vi "AWS Credentials Dialog.vi"(8 "error in (no error)":errorcluster) -> (0 "error out":errorcluster, 2 "Secret Access Key":string="fpHFy/9MTHgVK4Kfo+TPLrNeMAvaW8SEbrhzqAeY", 3 "Access Key ID":string="AKIAZ3CRVRJNHJHHHPO3")   [LabVIEW 2016, in "Data.S3.lvclass"]
uses:
  Data.S3/Data.S3.lvclass
  <vilib>/Platform/browser.llb/Open URL in Default Browser (string).vi
panel:
  in  "OK":bool caption="OK1"
  in  "HELP":bool caption="OK1"
  in  "Secret Access Key":string
  in  "Access Key ID":string
  out "String":string="Please enter your AWS credentials below:"
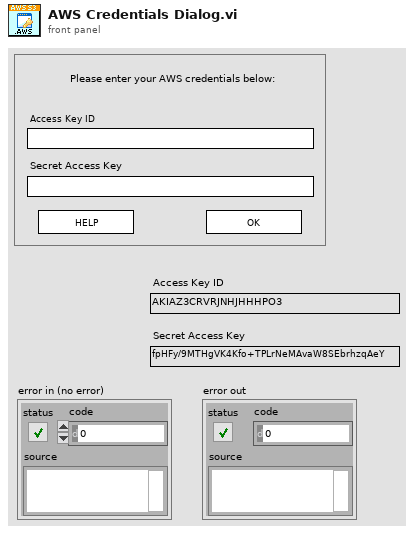
[diagram p1: front panel]
types:
  T1 = enum32{"Invalid", "Standard", "Closed", "Hidden", "Minimized", "Maximized"}
  T2 = enum32{"invalid app kind", "Development System", "Run Time System", "Student Edition", "Embedded LabVIEW", "Evaluation", "Custom"}
  T3 = cluster{"Core":cluster{"Current VI Reference":refnum<vi>, "Close Panel on Exit?":bool}, "Access Key ID":string, "Secret Access Key":string}
  T4 = cluster{"Current VI Reference":refnum<vi>, "Close Panel on Exit?":bool}
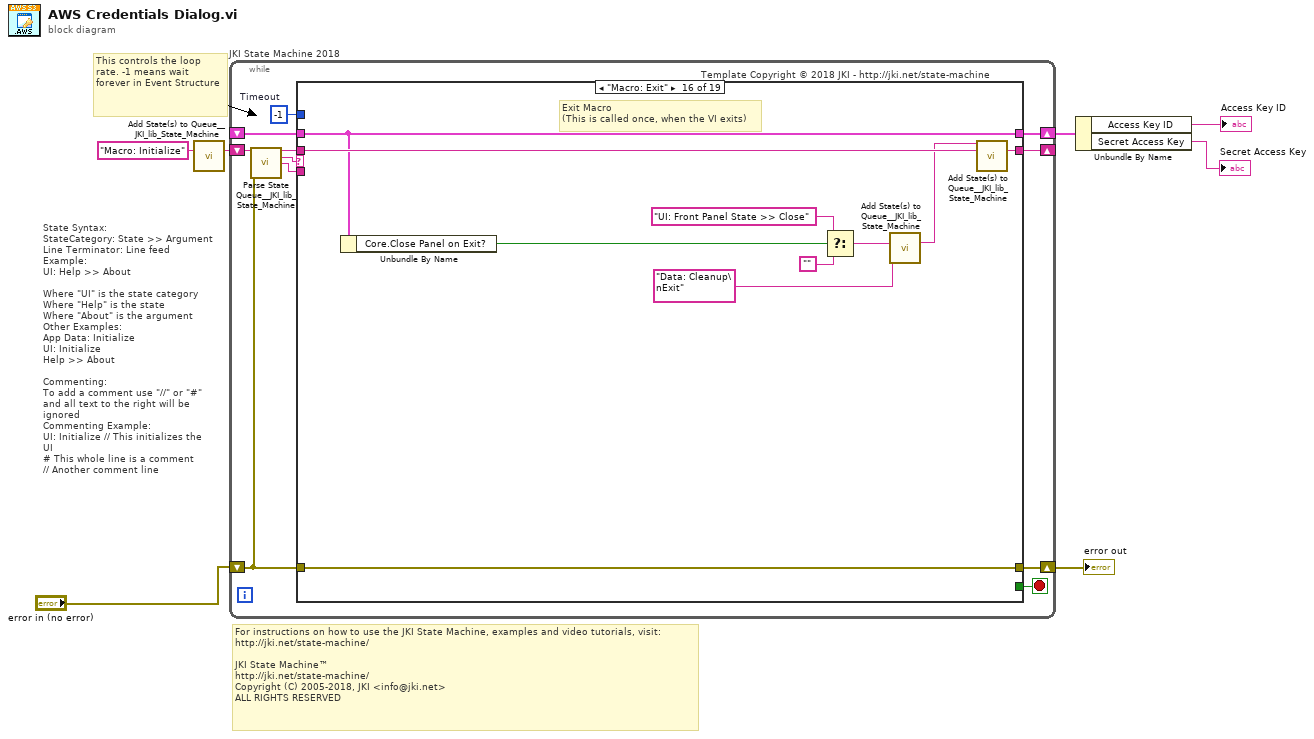
[diagram p0: block diagram]
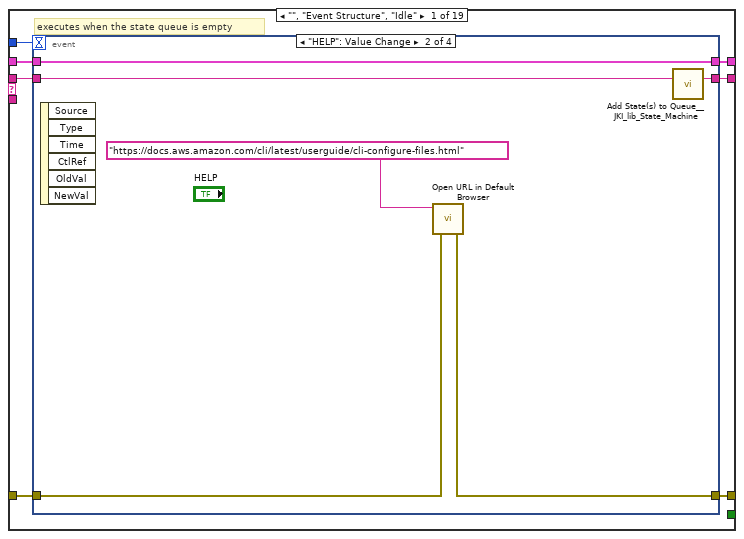
[diagram p2: hidden frame]
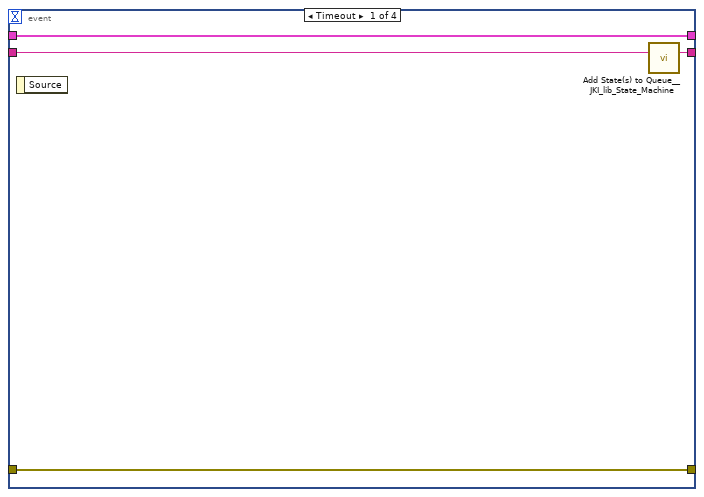
[diagram p3: hidden frame]
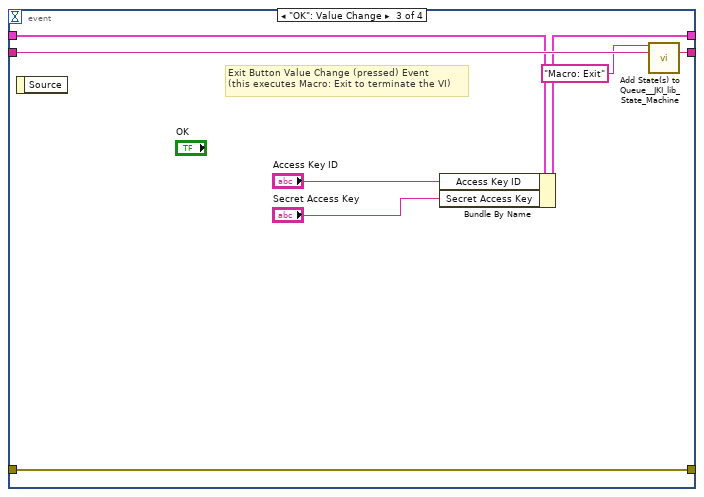
[diagram p4: hidden frame]
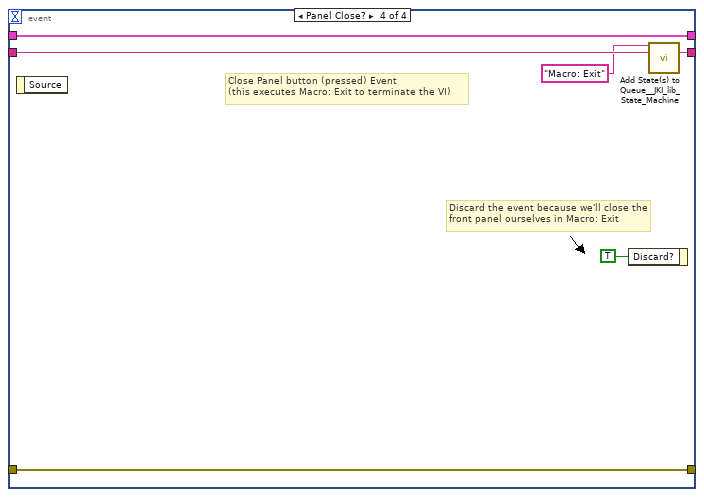
[diagram p5: hidden frame]
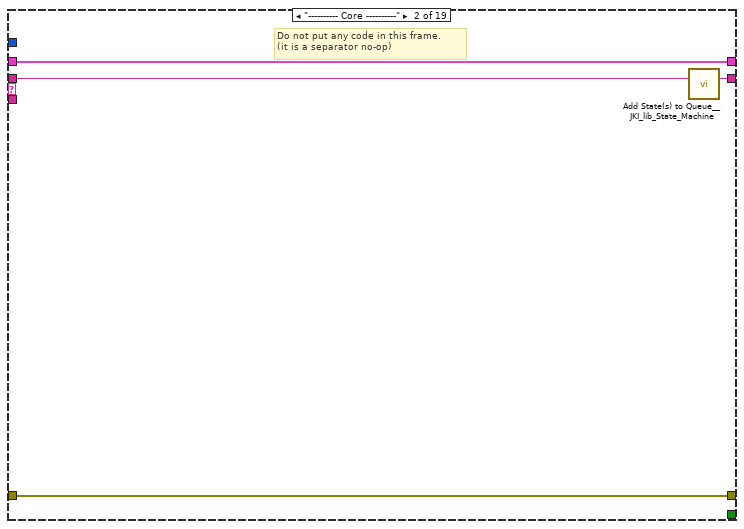
[diagram p6: hidden frame]
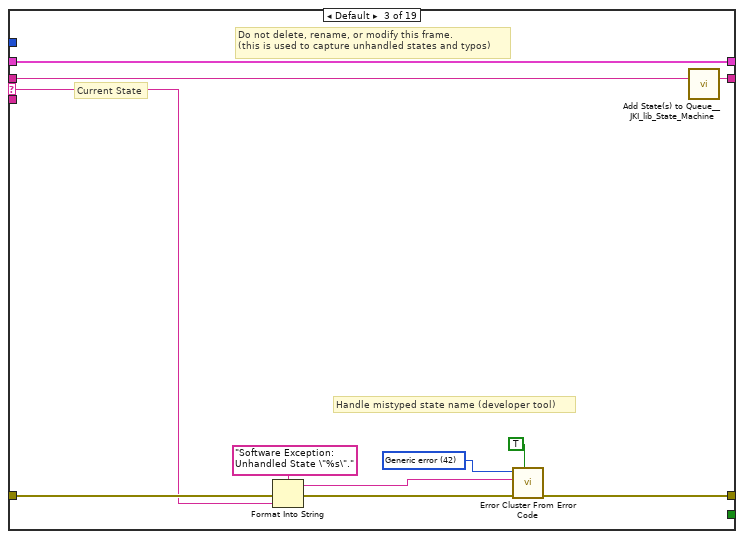
[diagram p7: hidden frame]
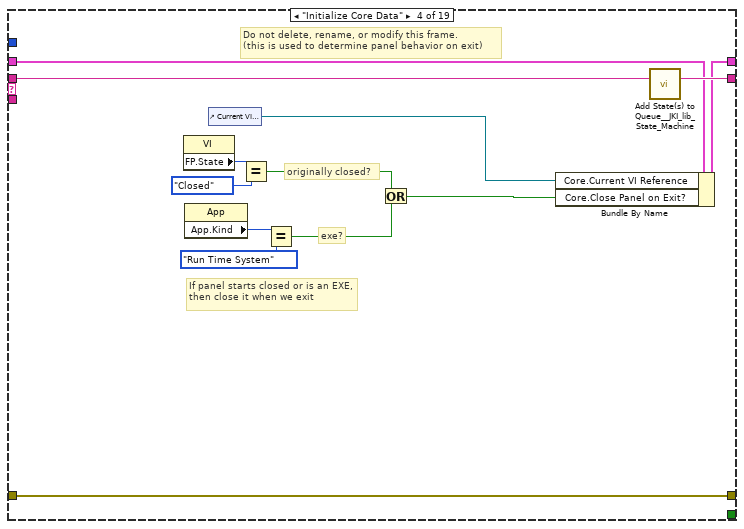
[diagram p8: hidden frame]
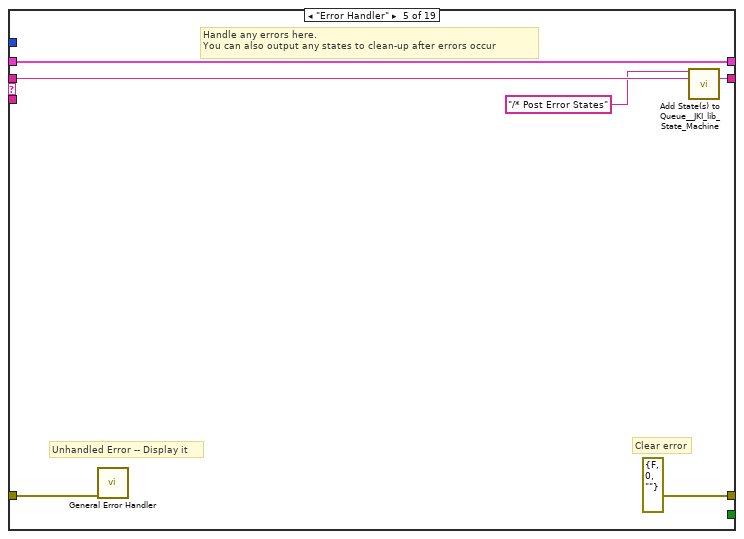
[diagram p9: hidden frame]
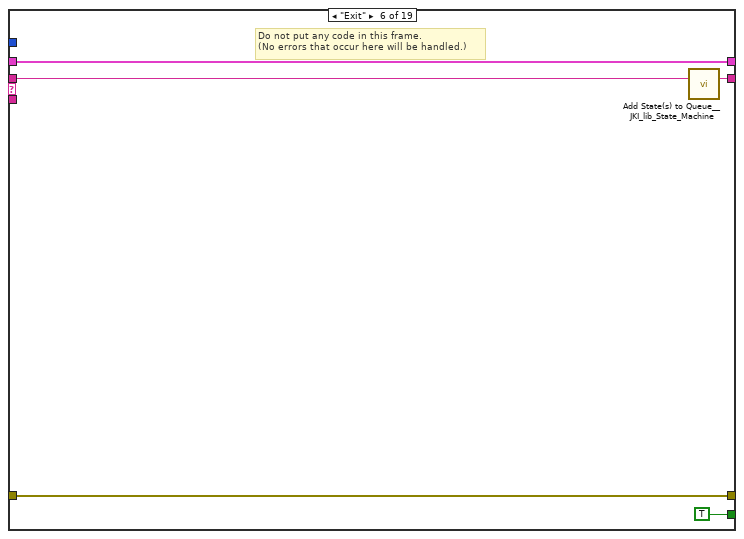
[diagram p10: hidden frame]
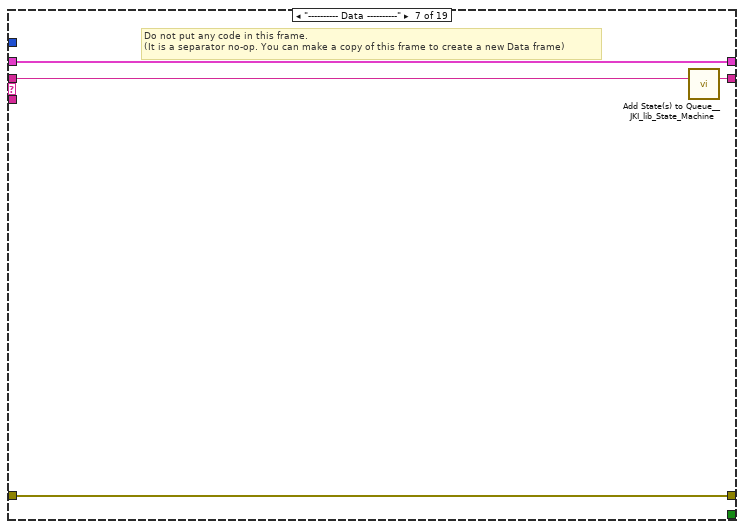
[diagram p11: hidden frame]
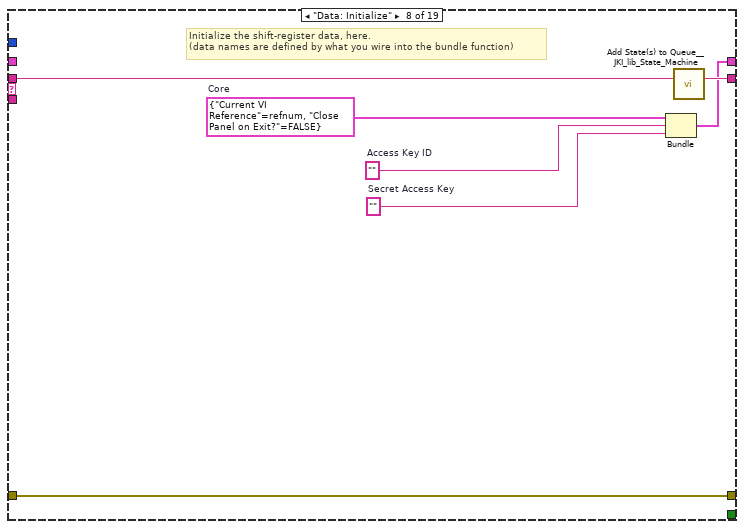
[diagram p12: hidden frame]
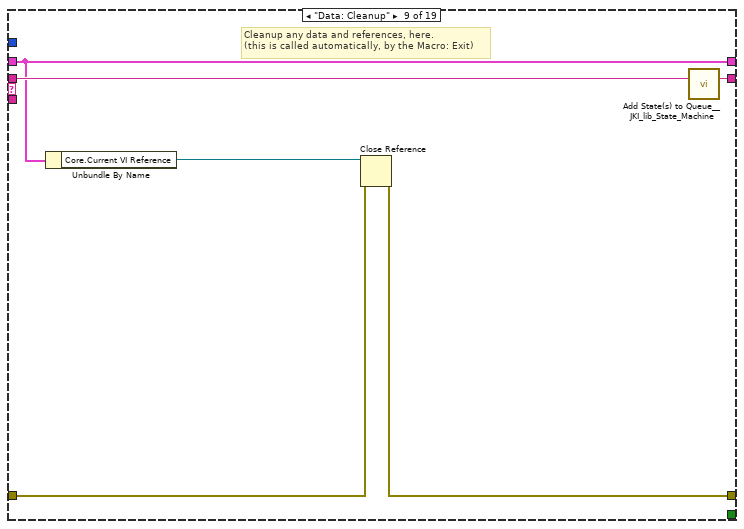
[diagram p13: hidden frame]
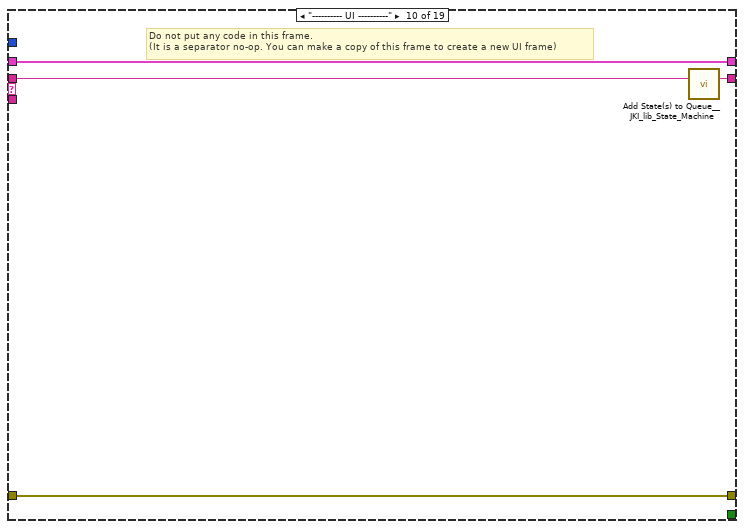
[diagram p14: hidden frame]
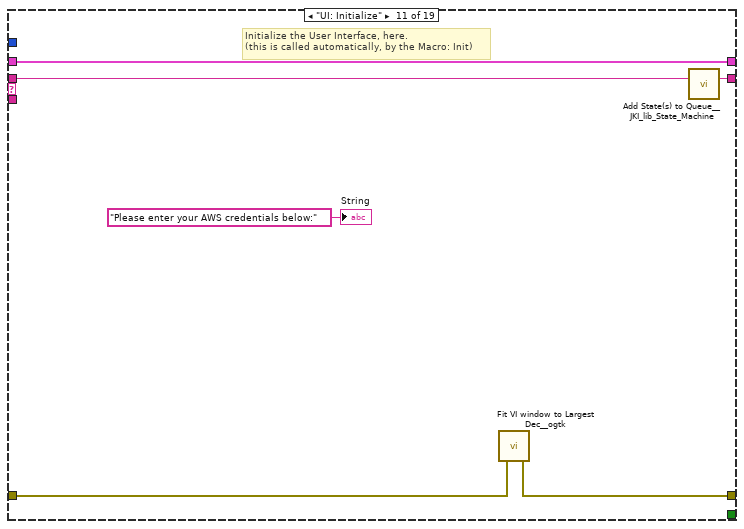
[diagram p15: hidden frame]
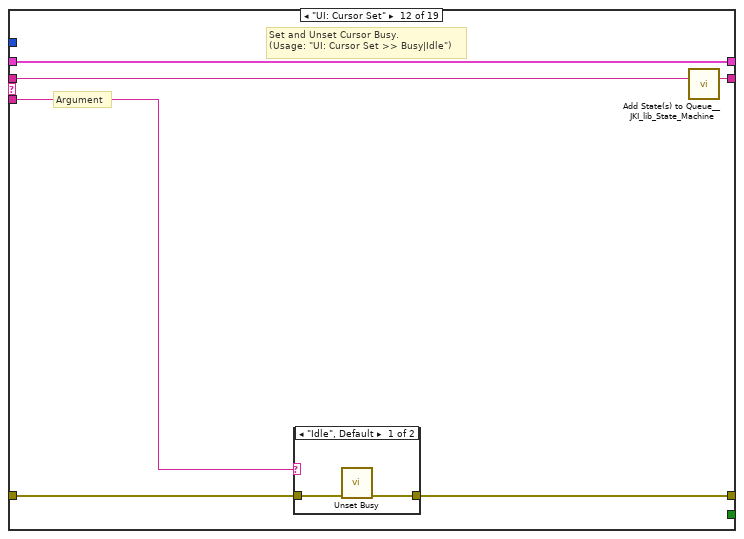
[diagram p16: hidden frame]
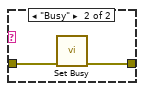
[diagram p17: hidden frame]
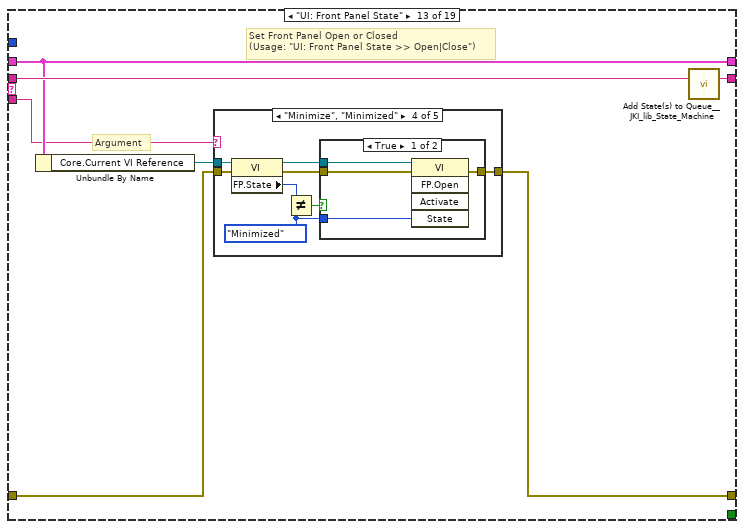
[diagram p18: hidden frame]
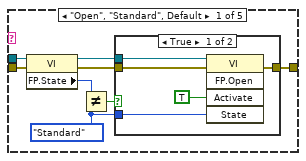
[diagram p19: hidden frame]
diagram:
  # "For instructions on how to use the JKI State Machine, examples and video tutorials, visit:\nhttp://jki.net/state-machine/\n\nJKI State Machine™\nhttp://jki.net/state-machine/\nCopyright (C) 2005-2018, JKI <info@jki.net>\nALL RIGHTS RESERVED"
  # "State Syntax:\nStateCategory: State >> Argument\nLine Terminator: Line feed\nExample:\nUI: Help >> About\n\nWhere \"UI\" is the state category\nWhere \"Help\" is the state\nWhere \"About\" is the argument\nOther Examples:\nApp Data: Initialize\nUI: Initialize\nHelp >> About\n\nCommenting:\nTo add a comment use \"//\" or \"#\" and all text to the right will be ignored\nCommenting Example:\nUI: Initialize // This initializes the UI\n# This whole line is a comment\n// Another comment line"
  # "This controls the loop rate. -1 means wait forever in Event Structure"
  n1 = call <vilib>:"Add State(s) to Queue__JKI_lib_State_Machine.vi"("State(s) in (\"\")"="Macro: Initialize") -> ("States Out"=w7:string)  [unwired: 14 in]
  n2 = while "JKI State Machine 2018" {
    shift-right: [w11] -> w3
    shift-left: _ -> [w10]
    shift-right: [w14] -> w5
    shift-left: "error in (no error)" -> [w8]
    shift-right: [w13] -> _
    shift-left: w7 -> [w15]
    stop <- w12 stop-if-true
    w9 = -1  # Timeout
    # "Template Copyright © 2018 JKI - http://jki.net/state-machine"
    n3 = call <vilib>:"Parse State Queue__JKI_lib_State_Machine.vi"("State Queue"=w15, "Error In (no error)"=w8) -> ("Remaining States"=w17:string, "Current State"=w18:string, "Arguments"=w16:string)  [unwired: 11 in]
    n4 = case shown="\"Macro: Exit\"" w18 {
      selector: w18 -> [_ _ w54 _ _ _ _ _ _ _ _ _ _ _ _ _ _ _ _]
      tunnel: w17 -> [w25 w53 w58 w77 w83 w88 w92 w99 w105 w109 w115 w121 w132 w201 w206 w216 w220 w224 w228]
      tunnel: w16 -> [_ _ _ _ _ _ _ _ _ _ _ w116 w126 _ _ _ _ _ _]
      tunnel: w10 -> [w23 w50 w56 w70 w80 w86 w89 _ w100 w106 w113 w119 w128 w198 w203 w213 w217 w221 w225]
      tunnel: [w22 w51 w60 w74 errorcluster {"status"=FALSE, "code"=0, "source"=""} ("error out") w85 w90 w96 w101 w107 w111 w117 w129 w199 w204 w214 w218 w222 w226] -> w14
      tunnel: w8 -> [w21 w51 w59 w74 w79 w85 w90 w96 w102 w107 w112 w118 w130 w199 w204 w214 w218 w222 w226]
      tunnel: [w24 w52 w57 w76 w82 w87 w91 w98 w104 w108 w114 w120 w131 w200 w205 w215 w219 w223 w227] -> w13
      tunnel: [_ _ _ _ _ TRUE _ _ _ _ _ _ _ _ _ _ _ _ _] -> w12
      tunnel: [w20 w50 w56 w75 w80 w86 w89 w97 w100 w106 w113 w119 w128 w198 w203 w213 w217 w221 w225] -> w11
      tunnel: w9 -> [w19 _ _ _ _ _ _ _ _ _ _ _ _ _ _ _ _ _ _]
      frame "", "Event Structure", "Idle" {
        # "executes when the state queue is empty"
        n5 = event shown="[1] \"HELP\": Value Change" {
          selector: _ -> [_ _ _ _]
          dyn-events: _ -> [_ _ _ _]
          timeout: w19 -> [_ _ _ _]
          tunnel: w25 -> [w29 w35 w43 w49]
          tunnel: [w28 w34 w42 w48] -> w24
          tunnel: w23 -> [w26 w33 w39 w46]
          tunnel: [w27 w31 w41 w47] -> w22
          tunnel: w21 -> [w27 w32 w41 w47]
          tunnel: [w26 w33 w38 w46] -> w20
          event Timeout {
            n6 = event-data() -> ()  [unwired: 1 in, 1 out]
            n7 = call <vilib>:"Add State(s) to Queue__JKI_lib_State_Machine.vi"("State(s) in (\"\")"=w29) -> ("States Out"=w28:string)  [unwired: 14 in]
          }
          event "HELP": Value Change {
            n8 = event-data() -> ()  [unwired: 1 in, 6 out]
            n9 = call-poly <vilib>:"Open URL in Default Browser.vi"("error in (no error)"=w32, "URL"="https://docs.aws.amazon.com/cli/latest/userguide/cli-configure-files.html") -> ("error out"=w31:errorcluster)  [unwired: 4 in, 1 out]
            n10 = call <vilib>:"Add State(s) to Queue__JKI_lib_State_Machine.vi"("State(s) in (\"\")"=w35) -> ("States Out"=w34:string)  [unwired: 14 in]
          }
          event "OK": Value Change {
            # "Exit Button Value Change (pressed) Event\n(this executes Macro: Exit to terminate the VI)"
            n11 = event-data() -> ()  [unwired: 1 in, 1 out]
            n12 = Bundle By Name(cluster=w39, "Access Key ID"="Access Key ID", "Secret Access Key"="Secret Access Key") -> (w38:T3)
            n13 = call <vilib>:"Add State(s) to Queue__JKI_lib_State_Machine.vi"("State(s) in Front (\"\")"="Macro: Exit", "State(s) in (\"\")"=w43) -> ("States Out"=w42:string)  [unwired: 13 in]
          }
          event Panel Close? {
            # "Discard the event because we'll close the front panel ourselves in Macro: Exit"
            # "Close Panel button (pressed) Event\n(this executes Macro: Exit to terminate the VI)"
            n14 = event-data() -> ()  [unwired: 1 in, 1 out]
            n15 = event-data("Discard?"=TRUE) -> ()  [unwired: 1 in, 1 out]
            n16 = call <vilib>:"Add State(s) to Queue__JKI_lib_State_Machine.vi"("State(s) in Front (\"\")"="Macro: Exit", "State(s) in (\"\")"=w49) -> ("States Out"=w48:string)  [unwired: 13 in]
          }
        }
      }
      frame "---------- Core ----------" {
        # "Do not put any code in this frame.\n(it is a separator no-op)"
        n17 = call <vilib>:"Add State(s) to Queue__JKI_lib_State_Machine.vi"("State(s) in (\"\")"=w53) -> ("States Out"=w52:string)  [unwired: 14 in]
      }
      frame Default {
        w63 = 42 items=["No error", "Argument error", "Memory is full", "Out of zone", "End of file", "File already open", "Generic file I/O error", "File not found", "File permission error", "Disk is full", "Duplicate path", "Too many files open", "System feature not enabled", "Resource file not found", "Cannot add resource", "Resource not found", "Image not found", "Image memory error", "Pen does not exist", "Config type invalid", "Config token not found", "Config parse error", "Config memory error", "Bad external code format", "Bad external code offset", "External code not present", "Null window", "Destroy window error", "Null menu", "Print aborted", "Bad print record", "Print driver error", "Windows error during printing", "Memory error during printing", "Print dialog error", "Generic print error", "Invalid device refnum", "Device not found", "Device parameter error", "Device unit error", "Cannot open device", "Device call aborted", "Generic error", "Cancelled by user", "Object ID too low", "Object ID too high", "Object not in heap", "Unknown heap", "Unknown object (invalid DefProc)", "Unknown object (DefProc not in table)", "Message out of range", "Invalid (null) method", "Unknown message", "Manager call not supported", "Bad address", "Network operation in progress", "Network operation timed out", "Connection is busy", "Network attribute not supported", "Network error", "Address in use", "System out of memory", "Connection aborted", "Connection refused", "Not connected", "Already connected", "Connection closed", "Initialization error (interapplication manager)", "Bad occurrence", "Wait on unbound occurrence handler", "Occurrence queue overflow", "Datalog type conflict", "Unused", "Unrecognized type (interapplication manager)", "Memory corrupt", "Failed to make temporary DLL", "Old CIN version", "Drag socket not found", "Failed to load drop-object", "Failed to register OLE object", "Failed to release OLE object", "Format specifier type mismatch", "Unknown format specifier", "Too few format specifiers", "Too many format specifiers", "Scan failed", "Newer CIN version", "Error converting to variant", "Runtime menu error", "Password tampered", "Variant attribute not found", "Incompatible variant data type", "Event data is not available", "Event Store is not present", "Occurrence is not found", "Event Queue is not created", "Event info is not available", "Refnum passed is NULL", "Error retrieving Class GUID", "Error retrieving CoClass GUID", "Error retrieving TypeLib GUID.", "Bad built application magic bytes.", "Specific driver is different from the specific driver associated with the Logical Name.", "There is no session opened to the class driver.", "Max Error", "MAX - Error with config objects", "MAX - Error loading configuration", "MAX - Group not supported"]
        # "Current State"
        # "Do not delete, rename, or modify this frame.\n(this is used to capture unhandled states and typos)"
        # "Handle mistyped state name (developer tool)"
        n18 = Format Into String(format string="Software Exception: Unhandled State \"%s\"." ("message"), error in=w59, w54) -> (resulting string=w62:string, error out=w61:errorcluster)  [unwired: 1 in]
        n19 = call <vilib>:"Error Cluster From Error Code.vi"("show call chain? (False)"=TRUE, "error in (no error)"=w61, "error message (\"\")"=w62, "error code (0)"=w63) -> ("error out"=w60:errorcluster)  [unwired: 5 in]
        n20 = call <vilib>:"Add State(s) to Queue__JKI_lib_State_Machine.vi"("State(s) in (\"\")"=w58) -> ("States Out"=w57:string)  [unwired: 14 in]
      }
      frame "Initialize Core Data" {
        # "Do not delete, rename, or modify this frame.\n(this is used to determine panel behavior on exit)"
        # "originally closed?"
        # "exe?"
        # "If panel starts closed or is an EXE, then close it when we exit"
        n21 = property class="VI"() -> ("FP.State"=w67:T1)  [unwired: 2 in, 2 out]
        n22 = property class="App"() -> ("App.Kind"=w73:T2)  [unwired: 2 in, 2 out]
        n23 = control-ref of="Current VI Reference"() -> (w68:refnum<vi>)
        n24 = Equal?(x=w67, y=T1."Closed" ("Front Panel Window:State")) -> (x = y?=w65:bool)
        n25 = Equal?(x=w73, y=T2."Run Time System" ("Application:Kind")) -> (x = y?=w71:bool)
        n26 = Or(x=w65, y=w71) -> (x .or. y?=w69:bool)
        n27 = Bundle By Name(cluster=w70, "Core.Current VI Reference"=w68, "Core.Close Panel on Exit?"=w69) -> (w75:T3)
        n28 = call <vilib>:"Add State(s) to Queue__JKI_lib_State_Machine.vi"("State(s) in (\"\")"=w77) -> ("States Out"=w76:string)  [unwired: 14 in]
      }
      frame "Error Handler" {
        # "Unhandled Error -- Display it"
        # "Handle any errors here.\nYou can also output any states to clean-up after errors occur"
        # "Clear error"
        n29 = call <vilib>:"General Error Handler.vi"("error in (no error)"=w79) -> ()  [unwired: 10 in, 5 out]
        n30 = call <vilib>:"Add State(s) to Queue__JKI_lib_State_Machine.vi"("State(s) in Front (\"\")"="/* Post Error States", "State(s) in (\"\")"=w83) -> ("States Out"=w82:string)  [unwired: 13 in]
      }
      frame "Exit" {
        # "Do not put any code in this frame.\n(No errors that occur here will be handled.)"
        n31 = call <vilib>:"Add State(s) to Queue__JKI_lib_State_Machine.vi"("State(s) in (\"\")"=w88) -> ("States Out"=w87:string)  [unwired: 14 in]
      }
      frame "---------- Data ----------" {
        # "Do not put any code in this frame.\n(It is a separator no-op. You can make a copy of this frame to create a new Data frame)"
        n32 = call <vilib>:"Add State(s) to Queue__JKI_lib_State_Machine.vi"("State(s) in (\"\")"=w92) -> ("States Out"=w91:string)  [unwired: 14 in]
      }
      frame "Data: Initialize" {
        w93 = ""  # Access Key ID
        w94 = T4 {"Current VI Reference"=refnum, "Close Panel on Exit?"=FALSE}  # Core
        w95 = ""  # Secret Access Key
        # "Initialize the shift-register data, here.\n(data names are defined by what you wire into the bundle function)"
        n33 = Bundle("Core"=w94, "Access Key ID"=w93, "Secret Access Key"=w95) -> (w97:T3)  [unwired: 1 in]
        n34 = call <vilib>:"Add State(s) to Queue__JKI_lib_State_Machine.vi"("State(s) in (\"\")"=w99) -> ("States Out"=w98:string)  [unwired: 14 in]
      }
      frame "Data: Cleanup" {
        # "Cleanup any data and references, here.\n(this is called automatically, by the Macro: Exit)"
        n35 = Unbundle By Name(w100) -> ("Core.Current VI Reference"=w103:refnum<vi>)
        n36 = Close Reference(reference=w103, error in (no error)=w102) -> (error out=w101:errorcluster)
        n37 = call <vilib>:"Add State(s) to Queue__JKI_lib_State_Machine.vi"("State(s) in (\"\")"=w105) -> ("States Out"=w104:string)  [unwired: 14 in]
      }
      frame "---------- UI ----------" {
        # "Do not put any code in this frame.\n(It is a separator no-op. You can make a copy of this frame to create a new UI frame)"
        n38 = call <vilib>:"Add State(s) to Queue__JKI_lib_State_Machine.vi"("State(s) in (\"\")"=w109) -> ("States Out"=w108:string)  [unwired: 14 in]
      }
      frame "UI: Initialize" {
        # "Initialize the User Interface, here.\n(this is called automatically, by the Macro: Init)"
        n39 = call <userlib>:"Fit VI window to Largest Dec__ogtk.vi"("error in (no error)"=w112) -> ("error out"=w111:errorcluster)  [unwired: 5 in, 1 out]
        n40 = call <vilib>:"Add State(s) to Queue__JKI_lib_State_Machine.vi"("State(s) in (\"\")"=w115) -> ("States Out"=w114:string)  [unwired: 14 in]
        "String" <- "Please enter your AWS credentials below:" ("String")
      }
      frame "UI: Cursor Set" {
        # "Argument"
        # "Set and Unset Cursor Busy.\n(Usage: \"UI: Cursor Set >> Busy|Idle\")"
        n41 = case shown="\"Idle\", Default" w116 {
          tunnel: w118 -> [w123 w125]
          tunnel: [w122 w124] -> w117
          frame "Idle", Default {
            n42 = call <vilib>:"Unset Busy.vi"("error in (no error)"=w123) -> ("error out"=w122:errorcluster)  [unwired: 10 in]
          }
          frame "Busy" {
            n43 = call <vilib>:"Set Busy.vi"("error in (no error)"=w125) -> ("error out"=w124:errorcluster)  [unwired: 9 in, 1 out]
          }
        }
        n44 = call <vilib>:"Add State(s) to Queue__JKI_lib_State_Machine.vi"("State(s) in (\"\")"=w121) -> ("States Out"=w120:string)  [unwired: 14 in]
      }
      frame "UI: Front Panel State" {
        # "Argument"
        # "Set Front Panel Open or Closed\n(Usage: \"UI: Front Panel State >> Open|Close\")"
        n45 = Unbundle By Name(w128) -> ("Core.Current VI Reference"=w127:refnum<vi>)
        n46 = case shown="\"Minimize\", \"Minimized\"" w126 {
          tunnel: w130 -> [w138 w153 w164 w177 w190]
          tunnel: [w140 w154 w166 w179 w192] -> w129
          tunnel: w127 -> [w139 w151 w165 w178 w191]
          frame "Open", "Standard", Default {
            w133 = T1."Standard" ("State")
            n47 = property class="VI"(reference=w139, error in=w138) -> (reference out=w136:refnum<vi>, error out=w137:errorcluster, "FP.State"=w135:T1)
            n48 = Not Equal?(x=w135, y=w133) -> (x != y?=w134:bool)
            n49 = case shown="True" w134 {
              tunnel: [w144 w146] -> w140
              tunnel: w137 -> [w143 w146]
              tunnel: w136 -> [w142 _]
              tunnel: w133 -> [w141 _]
              frame True {
                n50 = invoke class="VI" method="FP.Open"(reference=w142, error in=w143, "Activate"=TRUE, "State"=w141) -> (error out=w144:errorcluster)  [unwired: 1 in, 4 out]
              }
              frame False {
              }
            }
          }
          frame "Close", "Closed" {
            n51 = property class="VI"(reference=w151, error in=w153) -> (reference out=w150:refnum<vi>, error out=w152:errorcluster, "FP.State"=w148:T1)
            n52 = Not Equal?(x=w148, y=T1."Closed" ("Front Panel Window:State")) -> (x != y?=w147:bool)
            n53 = case shown="True" w147 {
              tunnel: [w155 w158] -> w154
              tunnel: w152 -> [w155 w157]
              tunnel: w150 -> [_ w156]
              frame False {
              }
              frame True {
                n54 = invoke class="VI" method="FP.Close"(reference=w156, error in=w157) -> (error out=w158:errorcluster)  [unwired: 1 in, 2 out]
              }
            }
          }
          frame "Hidden", "Hide" {
            w159 = T1."Hidden" ("State")
            n55 = property class="VI"(reference=w165, error in=w164) -> (reference out=w162:refnum<vi>, error out=w163:errorcluster, "FP.State"=w161:T1)
            n56 = Not Equal?(x=w161, y=w159) -> (x != y?=w160:bool)
            n57 = case shown="True" w160 {
              tunnel: [w170 w171] -> w166
              tunnel: w163 -> [w169 w171]
              tunnel: w162 -> [w168 _]
              tunnel: w159 -> [w167 _]
              frame True {
                n58 = invoke class="VI" method="FP.Open"(reference=w168, error in=w169, "State"=w167) -> (error out=w170:errorcluster)  [unwired: 2 in, 4 out]
              }
              frame False {
              }
            }
          }
          frame "Minimize", "Minimized" {
            w172 = T1."Minimized" ("State")
            n59 = property class="VI"(reference=w178, error in=w177) -> (reference out=w175:refnum<vi>, error out=w176:errorcluster, "FP.State"=w174:T1)
            n60 = Not Equal?(x=w174, y=w172) -> (x != y?=w173:bool)
            n61 = case shown="True" w173 {
              tunnel: [w183 w184] -> w179
              tunnel: w176 -> [w182 w184]
              tunnel: w175 -> [w181 _]
              tunnel: w172 -> [w180 _]
              frame True {
                n62 = invoke class="VI" method="FP.Open"(reference=w181, error in=w182, "State"=w180) -> (error out=w183:errorcluster)  [unwired: 2 in, 4 out]
              }
              frame False {
              }
            }
          }
          frame "Maximize", "Maximized" {
            w185 = T1."Maximized" ("State")
            n63 = property class="VI"(reference=w191, error in=w190) -> (reference out=w188:refnum<vi>, error out=w189:errorcluster, "FP.State"=w187:T1)
            n64 = Not Equal?(x=w187, y=w185) -> (x != y?=w186:bool)
            n65 = case shown="True" w186 {
              tunnel: [w196 w197] -> w192
              tunnel: w189 -> [w195 w197]
              tunnel: w188 -> [w194 _]
              tunnel: w185 -> [w193 _]
              frame True {
                n66 = invoke class="VI" method="FP.Open"(reference=w194, error in=w195, "State"=w193) -> (error out=w196:errorcluster)  [unwired: 2 in, 4 out]
              }
              frame False {
              }
            }
          }
        }
        n67 = call <vilib>:"Add State(s) to Queue__JKI_lib_State_Machine.vi"("State(s) in (\"\")"=w132) -> ("States Out"=w131:string)  [unwired: 14 in]
      }
      frame "---------- Macro ----------" {
        # "Do not put any code in this frame.\n(It is a separator no-op. You can make a copy of this frame to create a new Macro frame)"
        n68 = call <vilib>:"Add State(s) to Queue__JKI_lib_State_Machine.vi"("State(s) in (\"\")"=w201) -> ("States Out"=w200:string)  [unwired: 14 in]
      }
      frame "Macro: Initialize" {
        w202 = "Data: Initialize\nInitialize Core Data\nUI: Initialize\nUI: Front Panel State >> Open"  # Data: Initialize Initialize Core Data UI: Initialize UI: Front Panel State >> Open
        # "Initialization Macro\n(This is called once, when the VI starts)"
        n69 = call <vilib>:"Add State(s) to Queue__JKI_lib_State_Machine.vi"("State(s) in Front (\"\")"=w202, "State(s) in (\"\")"=w206) -> ("States Out"=w205:string)  [unwired: 13 in]
      }
      frame "Macro: Exit" {
        # "Exit Macro\n(This is called once, when the VI exits)"
        n70 = Unbundle By Name(w213) -> ("Core.Close Panel on Exit?"=w212:bool)
        n71 = Select(t="UI: Front Panel State >> Close", s=w212, f="") -> (s? t:f=w209:string)
        n72 = call <vilib>:"Add State(s) to Queue__JKI_lib_State_Machine.vi"("State(s) in (\"\")"=w209, "State(s) at Back (\"\")"="Data: Cleanup\nExit") -> ("States Out"=w207:string)  [unwired: 13 in]
        n73 = call <vilib>:"Add State(s) to Queue__JKI_lib_State_Machine.vi"("State(s) in Front (\"\")"=w207, "State(s) in (\"\")"=w216) -> ("States Out"=w215:string)  [unwired: 13 in]
      }
      frame "---------- New Category ----------" {
        # "Template Separator\n(You can make a copy of, or modify, this frame)"
        n74 = call <vilib>:"Add State(s) to Queue__JKI_lib_State_Machine.vi"("State(s) in (\"\")"=w220) -> ("States Out"=w219:string)  [unwired: 14 in]
      }
      frame "New Category: 1" {
        # "Your code here.\n(You can make a copy of, or modify, this frame)"
        n75 = call <vilib>:"Add State(s) to Queue__JKI_lib_State_Machine.vi"("State(s) in (\"\")"=w224) -> ("States Out"=w223:string)  [unwired: 14 in]
      }
      frame "New Category: 2" {
        # "Your code here.\n(You can make a copy of, or modify, this frame)"
        n76 = call <vilib>:"Add State(s) to Queue__JKI_lib_State_Machine.vi"("State(s) in (\"\")"=w228) -> ("States Out"=w227:string)  [unwired: 14 in]
      }
    }
  }
  "error out" <- w5
  n77 = Unbundle By Name(w3) -> ("Access Key ID"=→"Access Key ID":string, "Secret Access Key"=→"Secret Access Key":string)
